vi "read_params.vi"(8 "error in (no error)":errorcluster, 11 "Ridge in":refnum<class "Ridge.lvclass">) -> (0 "error out":errorcluster, 2 "params":T1={"alpha"={"alpha_type"="float", "alpha_float"=1.0, "alpha_list"=[]}, "fit_intercept"=TRUE, "normalize"=FALSE, "copy_X"=TRUE, "max_iter"={"max_iter_type"="None", "max_iter_int"=0.0}, "tol"=0.001, "solver"="auto", "random_state"=0.0}, 3 "Ridge out":refnum<class "Ridge.lvclass">)   [LabVIEW 2020, in "Ridge.lvclass"]
uses:
  Ridge.lvclass
  Controls/ridge_params.ctl
  Ridge.lvclass/Ridge.ctl
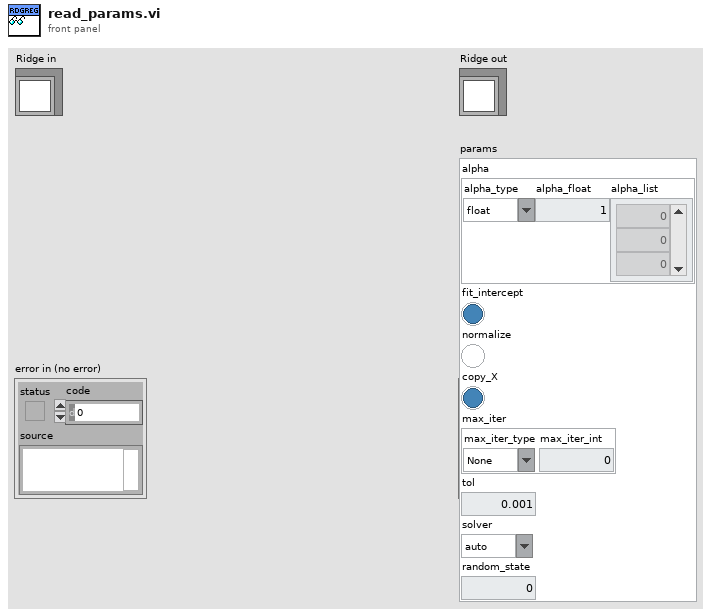
[diagram p1: front panel]
types:
  T1 = typedef "ridge_params.ctl" = cluster{"alpha":cluster{"alpha_type":string, "alpha_float":dbl, "alpha_list":dbl[]}, "fit_intercept":bool, "normalize":bool, "copy_X":bool, "max_iter":cluster{"max_iter_type":string, "max_iter_int":dbl}, "tol":dbl, "solver":string, "random_state":dbl}
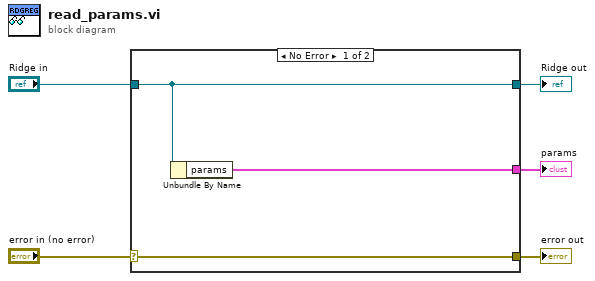
[diagram p0: block diagram]
diagram:
  n1 = case shown="No Error" "error in (no error)" {
    selector: "error in (no error)" -> [w8 w9]
    tunnel: [w8 w9] -> w4
    tunnel: [w7 w10] -> w2
    tunnel: "Ridge in" -> [w7 w10]
    tunnel: [w6 _] -> w1
    frame No Error {
      n2 = Unbundle By Name(w7) -> ("params"=w6:T1)
    }
    frame Error {
    }
  }
  "error out" <- w4
  "Ridge out" <- w2
  "params" <- w1
